vi "set Timeout.vi"(8 "error in (no error)":errorcluster, 10 "timeout in ms (-1:never)":i32=-1, 11 "REx Command - Root in":refnum<class "REx Command - Root.lvclass">) -> (0 "error out":errorcluster, 3 "REx Command - Root out":refnum<class "REx Command - Root.lvclass">)   [LabVIEW 2012, in "REx.lvlib" / "REx Command - Root.lvclass"]
uses:
  REx Command - Root.lvclass
  REx Command - Root.lvclass/REx Command - Root.ctl
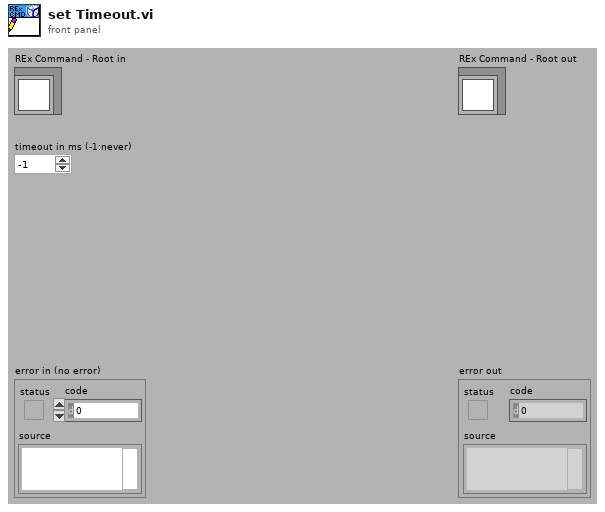
[diagram p1: front panel]
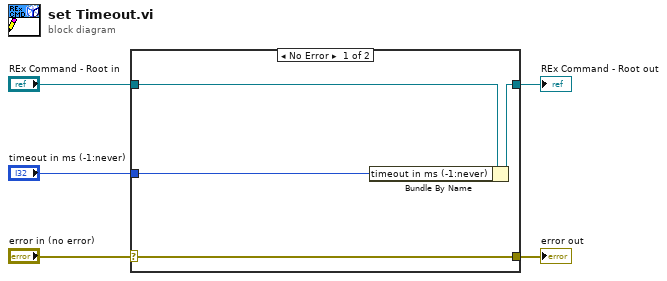
[diagram p0: block diagram]
diagram:
  n1 = case shown="No Error" "error in (no error)" {
    selector: "error in (no error)" -> [w9 w10]
    tunnel: [w9 w10] -> w4
    tunnel: [w7 w11] -> w2
    tunnel: "REx Command - Root in" -> [w8 w11]
    tunnel: "timeout in ms (-1:never)" -> [w6 _]
    frame No Error {
      n2 = Bundle By Name(cluster=w8, "timeout in ms (-1:never)"=w6) -> (w7:refnum<class "REx Command - Root.lvclass">)
    }
    frame Error {
    }
  }
  "error out" <- w4
  "REx Command - Root out" <- w2
